vi "Fluigent_Pressure_Fluctuation_KLT.vi"() -> ()   [LabVIEW 2020]
uses:
  <vilib>/DAQmx/read.llb/DAQmx Read (Analog 1D Wfm NChan NSamp).vi
  <userlib>/Fluigent/Fluigent MFCS/FluigentMFCS_Full.llb/MFCS_EZ Detect.vi
  <userlib>/Fluigent/Fluigent MFCS/FluigentMFCS_Full.llb/MFCS_EZ Initialization.vi
  <vilib>/DAQmx/create/channels.llb/DAQmx Create Channel (AI-Voltage-Basic).vi
  <vilib>/DAQmx/configure/timing.llb/DAQmx Timing (Sample Clock).vi
  <vilib>/Waveform/WDTOps.llb/WDT Get XY Value DBL.vi
  <userlib>/Fluigent/Fluigent MFCS/FluigentMFCS_Full.llb/MFCS_EZ Read All Channels Pressure.vi
  <vilib>/DAQmx/miscellaneous.llb/DAQmx Fill In Error Info.vi
  <userlib>/Fluigent/Fluigent MFCS/FluigentMFCS_Full.llb/MFCS_EZ Close.vi
  <vilib>/measure/NI_MABase.lvlib
panel:
  out "Finished":bool
  out "Time Elapsed (Min)":cluster{dbl, dbl}(slide)={5.0, 0.0} scale=0.0..5.0 scale format="%#_2g"
  out "Dev1 Samples":i32
  out "Running":bool
  in  "sampling info":cluster{"Fs":dbl, "#s":dbl}
  in  "Fs":dbl
  in  "Time (min)":dbl(knob)=5.0 min=0.1 max=5.0 step=0.1 scale=0.0..5.0 scale format="%#_2g"
  in  "Index File Labels Fluigent System":string[](array[string])=["1000", "nobody", "test", "1", "1", "junk"]
  out "Analog File Name Fluigent":string="C:\\yurong\\141104_12_31_1104"
  in  "Path for files Fluigent System":path=path "C:/Users/kkg5246/Desktop/Research/Fluigent Recordings"
  out "Current Voltage (V)":dbl
  out "Current Pressure (mmHg)":dbl
  out "Actual Pressure":dbl[](graph)
  out "Theoretical Pressure Waveform":waveform(dbl)(graph)={"t0"=timestamp(15 s since 1904-01-01), "dt"=0.001, "Y"=[]}
  in  "Voltage Conversion Factor":dbl=100.0 caption="Voltage Conversion Factor (1 V = x mmHg)" format="%0.2f"
  in  "Duty Cycle (%)":dbl=50.0 format="%0.2f"
  in  "Offset":dbl=250.0 format="%0.2p"
  in  "Reset Signal ?":bool
  in  "Signal Type":T1(ring)
  in  "Frequency (Hz)":dbl=5.0 format="%0.2p"
  in  "Amplitude (mmHg)":dbl=0.25 format="%0.2p"
  in  "Phase":dbl format="%0.2f"
  out "Phase out":dbl=180.0000000002135 format="%0.2f"
  in  "Stop":bool
  out "Waveform Chart":waveform(dbl)(graph)
  out "Pressure":dbl[](graph)=[0.00694105110600887]
  in  "physical channels":tag="Dev1/ai0"
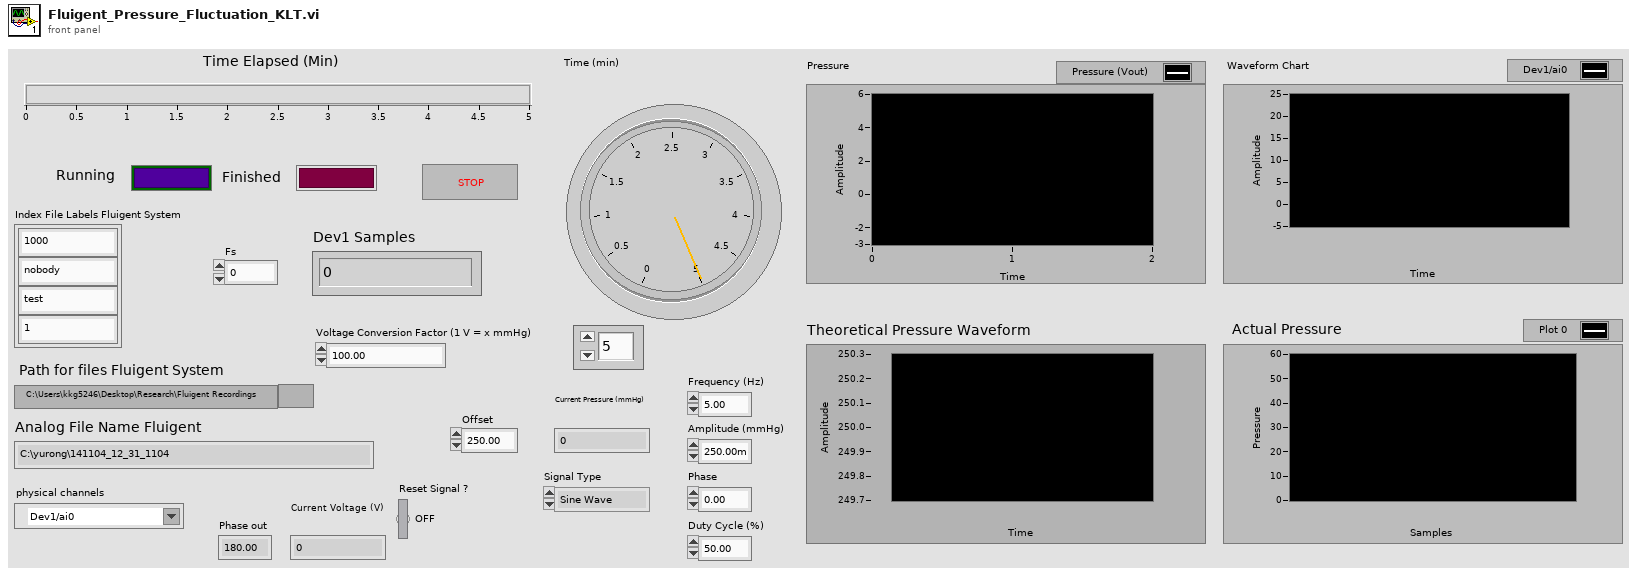
[diagram p1: front panel]
types:
  T1 = enum16{"Sine Wave", "Triangle Wave", "Square Wave", "Sawtooth Wave"}
  T2 = enum16{"open", "open or create", "create or replace", "create", "open (read-only)"}
  T3 = typedef "_EZmfcsSN.ctl" = u16
  T4 = typedef "_mfcs_EZ_handle.ctl" = u64
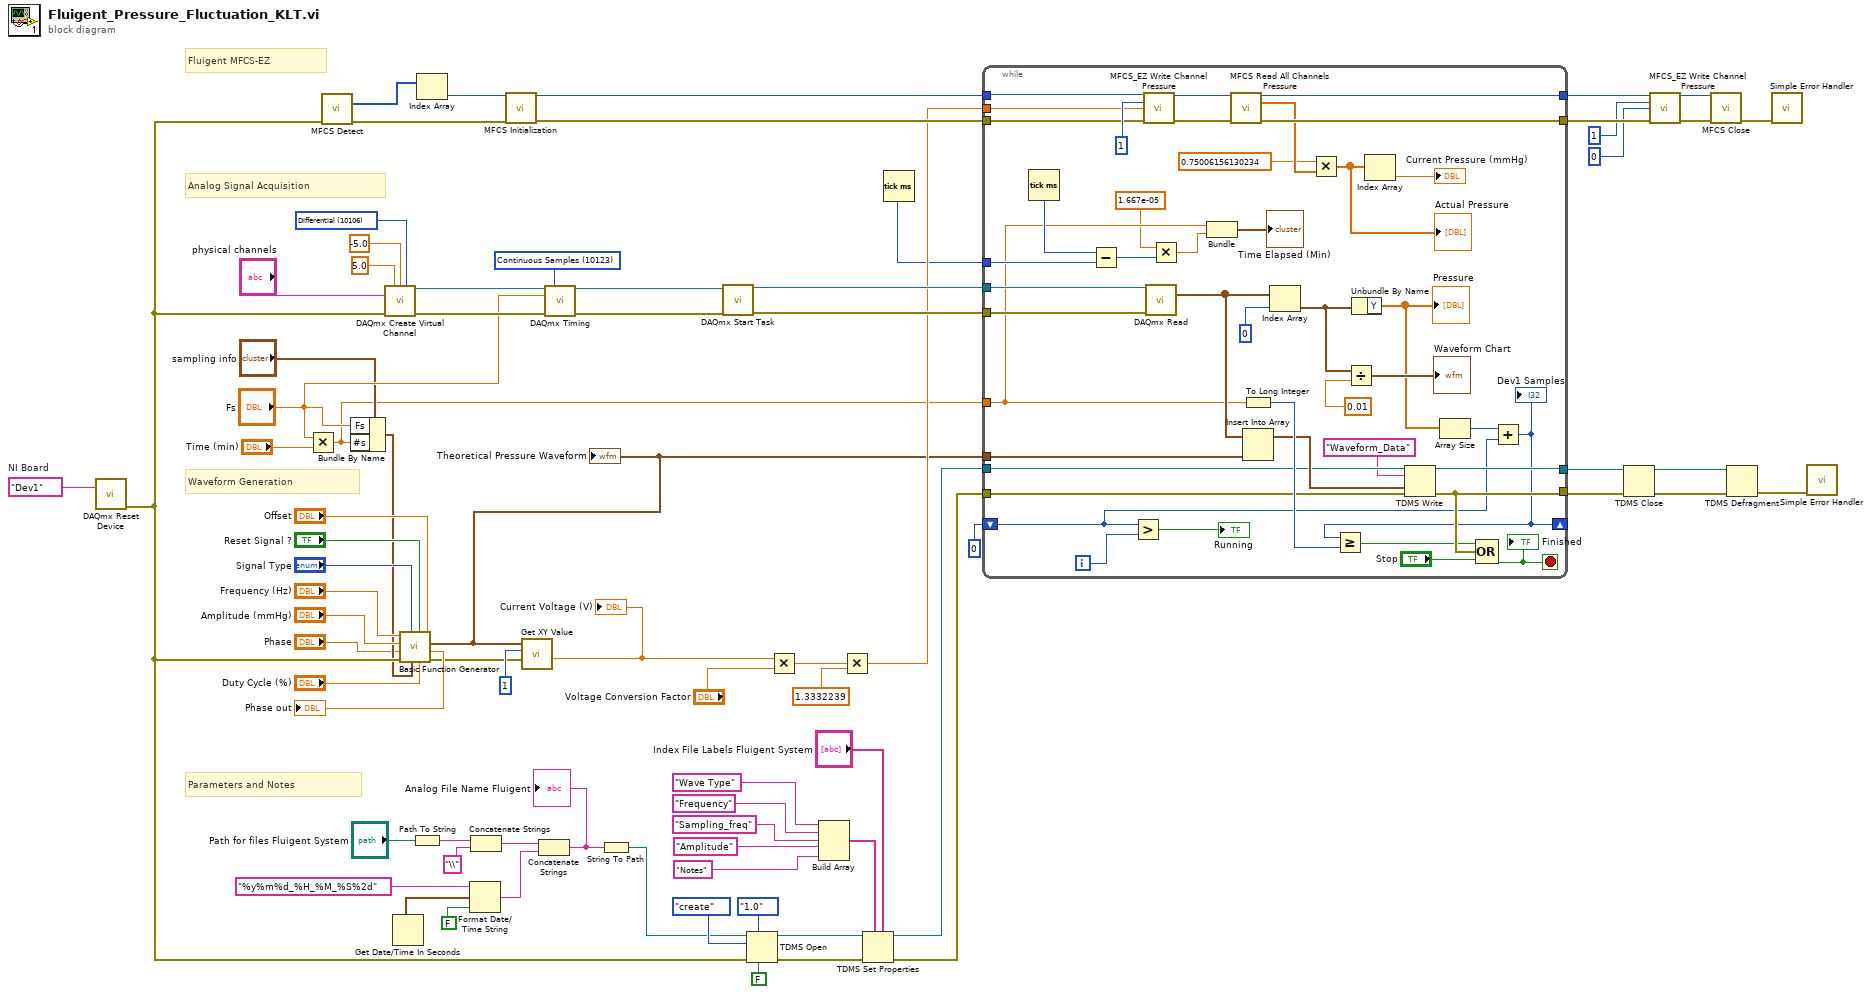
[diagram p0: block diagram]
diagram:
  w15 = tag "Dev1"  # NI Board
  w72 = 10106 items=["default"=-1, "RSE"=10083, "NRSE"=10078, "Differential"=10106, "Pseudodifferential"=12529] ("input terminal configuration")
  w76 = 10123 items=["Finite Samples"=10178, "Continuous Samples"=10123, "Hardware Timed Single Point"=12522] ("sample mode")
  # "Parameters and Notes"
  # "Waveform Generation"
  # "Analog Signal Acquisition"
  # "Fluigent MFCS-EZ"
  n1 = call <vilib>:"DAQmx Reset Device.vi"("device in"=w15) -> ("error out"=w14:errorcluster)  [unwired: 14 in]
  n2 = Multiply(x="Fs", y="Time (min)") -> (x*y=w5:dbl)
  n3 = call-poly <userlib>:"MFCS Detect.vi"("error in (no error)"=w14) -> ("[SN MFCS_EZ]"=w66:T3[], "error out"=w64:errorcluster)  [unwired: 13 in]
  n4 = Bundle By Name ("sampling info")(cluster="sampling info", "Fs"="Fs", "#s"=w5) -> (w12:cluster{"Fs":dbl, "#s":dbl})
  n5 = call-poly <vilib>:"DAQmx Create Virtual Channel.vi"("maximum value"=5.0, "minimum value"=-5.0, "input terminal configuration"=w72, "physical channels"="physical channels", "error in"=w14) -> ("task out"=w77:refnum<k21>, "error out"=w75:errorcluster)  [unwired: 4 in, 5 out]
  n6 = Get Date/Time In Seconds() -> (seconds since 1Jan1904=w52:timestamp)
  n7 = call <vilib>:"Basic Function Generator.vi"("offset"="Offset", "square wave duty cycle (%)"="Duty Cycle (%)", "reset signal"="Reset Signal ?", "sampling info"=w12, "signal type"="Signal Type", "error in (no error)"=w14, "phase"="Phase", "amplitude"="Amplitude (mmHg)", "frequency"="Frequency (Hz)") -> ("error out"=w13:errorcluster, "phase out"=→"Phase out":dbl, "signal out"=w2:waveform(dbl))
  "Theoretical Pressure Waveform" <- w2
  n8 = Path To String(path="Path for files Fluigent System") -> (string=w37:string)
  n9 = Index Array(array=w66) -> (element=w65:T3)  [unwired: 1 in]
  n10 = Format Date/Time String(time format string (%c)="%y%m%d_%H_%M_%S%2d", seconds (now)=w52, UTC format=FALSE) -> (date/time string=w49:string)
  n11 = Concatenate Strings(w37, "\\" ("string")) -> (w50:string)
  n12 = call-poly <userlib>:"MFCS Initialization.vi"("SN MFCS_EZ"=w65, "error in (no error)"=w64) -> ("MFCS_EZ_out"=w60:T4, "error out"=w59:errorcluster)  [unwired: 10 in, 2 out]
  n13 = call-poly <vilib>:"Get XY Value.vi"("error in (no error)"=w13, "Y position format"=1, "waveform in"=w2) -> ("Y value"=w16:dbl)  [unwired: 4 in, 4 out]
  "Current Voltage (V)" <- w16
  n14 = Concatenate Strings(w50, w49) -> (w48:string)
  "Analog File Name Fluigent" <- w48
  n15 = call-poly <vilib>:"DAQmx Timing.vi"("task/channels in"=w77, "sample mode"=w76, "rate"="Fs", "error in"=w75) -> ("task out"=w70:refnum<k21>, "error out"=w69:errorcluster)  [unwired: 3 in, 7 out]
  n16 = String To Path(string=w48) -> (path=w44:path)
  n17 = call <vilib>:"DAQmx Start Task.vi"("task/channels in"=w70, "error in"=w69) -> ("task out"=w68:refnum<k21>, "error out"=w67:errorcluster)  [unwired: 12 out]
  n18 = TDMS Open(6:FALSE ("disable buffering? (T)"), 7:enum16{"1.0", "2.0"}."1.0" ("file format version (2.0)"), 8:w14, 10:T2."create" ("operation (0:open)"), 11:w44) -> (0:w43:errorcluster, 3:w35:refnum<k34>)  [unwired: 2 in]
  n19 = Multiply(x=w16, y="Voltage Conversion Factor") -> (x*y=w28:dbl)
  n20 = Build Array("Wave Type", "Frequency", "Sampling_freq", "Amplitude", "Notes") -> (w38:string[])
  n21 = Multiply(x=w28, y=1.3332239) -> (x*y=w17:dbl)
  n22 = TDMS Set Properties(5:"Index File Labels Fluigent System", 7:w38, 8:w43, 11:w35) -> (0:w33:errorcluster, 3:w30:refnum<k34>)  [unwired: 4 out]
  n23 = Tick Count (ms)() -> (millisecond timer value=w1:u32)
  n24 = while {
    tunnel: w68 -> [w116]
    tunnel: w67 -> [w111]
    tunnel: w60 -> [w112]
    tunnel: w59 -> [w110]
    tunnel: [w109] -> w58
    tunnel: [w108] -> w55
    tunnel: w33 -> [w89]
    tunnel: [w100] -> w31
    tunnel: w30 -> [w87]
    tunnel: w17 -> [w103]
    tunnel: w2 -> [w90]
    tunnel: [w102] -> w8
    shift-right: [w92] -> _
    shift-left: 0 -> [w93]
    tunnel: w5 -> [w81]
    tunnel: w1 -> [w83]
    i -> [w98]
    stop <- w78 stop-if-true
    n25 = Tick Count (ms)() -> (millisecond timer value=w84:u32)
    n26 = Subtract(x=w84, y=w83) -> (x-y=w80:u32)
    n27 = Greater?(x=w93, y=w98) -> (0:→"Running":bool)
    n28 = call <userlib>:"MFCS_EZ Write Channel Pressure.vi"("MFCS_EZ"=w112, "Channel Number (default=1)"=1, "Pressure (mBar)"=w103, "error in (no error)"=w110) -> ("MFCS_EZ out"=w114:T4, "error out"=w115:errorcluster)  [unwired: 10 in]
    n29 = call-poly <vilib>:"DAQmx Read.vi"("task/channels in"=w116, "error in"=w111) -> ("data"=w91:waveform(dbl)[])  [unwired: 1 in, 12 out]
    n30 = Multiply(x=1.667e-05, y=w80) -> (x*y=w85:dbl)
    n31 = Bundle(w81, w85) -> (→"Time Elapsed (Min)":cluster{dbl, dbl})  [unwired: 1 in]
    n32 = call-poly <userlib>:"MFCS Read All Channels Pressure.vi"("MFCS_EZ"=w114, "error in (no error)"=w115) -> ("MFCS_EZ out"=w108:T4, "All Channels Pressure"=w107:dbl[], "error out"=w109:errorcluster)  [unwired: 11 in]
    n33 = To Long Integer(number=w81) -> (32bit integer=w97:i32)
    n34 = Insert Into Array(array=w91, new element=w90) -> (w88:waveform(dbl)[])  [unwired: 1 in]
    n35 = Index Array "Index Array"(array=w91, index=0 ("index (row)")) -> (element=w117:waveform(dbl))
    n36 = Multiply(x=0.75006156130234, y=w107) -> (x*y=w105:dbl[])
    "Actual Pressure" <- w105
    n37 = Divide(x=w117, y=0.01) -> (x/y=→"Waveform Chart":waveform(dbl))
    n38 = Unbundle By Name(w117) -> ("Y"=w95:dbl[])
    "Pressure" <- w95
    n39 = Index Array(array=w105) -> (element=→"Current Pressure (mmHg)":dbl)  [unwired: 1 in]
    n40 = TDMS Write(0:w87, 5:"Waveform_Data" ("string"), 9:w88, 11:w89) -> (4:w102:refnum<k34>, 15:w100:errorcluster)  [unwired: 2 in, 2 out]
    n41 = Array Size(array=w95) -> (size(s)=w94:i32)
    n42 = Add(x=w94, y=w93) -> (x+y=w92:i32)
    "Dev1 Samples" <- w92
    n43 = Greater Or Equal?(x=w92, y=w97) -> (x >= y?=w96:bool)
    n44 = Compound Arithmetic op=OR(w96, w100, "Stop") -> (w78:bool)
    "Finished" <- w78
  }
  n45 = TDMS Close(8:w31, 11:w8) -> (0:w32:errorcluster, 3:w3:path)
  n46 = call <userlib>:"MFCS_EZ Write Channel Pressure.vi"("MFCS_EZ"=w55, "Channel Number (default=1)"=1, "Pressure (mBar)"=0, "error in (no error)"=w58) -> ("MFCS_EZ out"=w61:T4, "error out"=w62:errorcluster)  [unwired: 10 in]
  n47 = call-poly <userlib>:"MFCS Close.vi"("MFCS_EZ"=w61, "error in (no error)"=w62) -> ("error out"=w63:errorcluster)  [unwired: 13 in]
  n48 = TDMS Defragment(4:w32, 7:w3) -> (0:w4:errorcluster)
  n49 = call <vilib>:"Simple Error Handler.vi"("error in (no error)"=w63) -> ()  [unwired: 4 in, 5 out]
  n50 = call <vilib>:"Simple Error Handler.vi"("error in (no error)"=w4) -> ()  [unwired: 4 in, 5 out]
